vi "Copy of Pulse Train Generation TIO.vi"(8 "error in":errorcluster) -> (0 "error out":errorcluster, 3 "Pulse Generation Task ID's Out":u32[](array[numeric]) format="%.0x")   [LabVIEW 2009]
uses:
  Acquisition Settings.vi
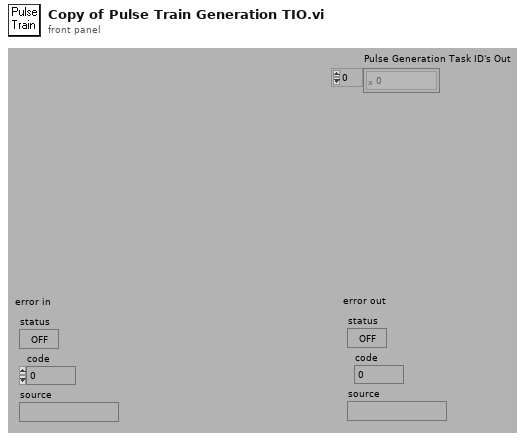
[diagram p1: front panel]
types:
  T1 = cluster{"Name":string, "Device Number":i16, "Counter Number":i16, "Pulse Spec 1 (Clocks)":u32, "Pulse Spec 2 (Clocks)":u32, "Signal Routing Configuration":i16, "Inverted":bool}[]
  T2 = cluster{"Name":string, "Signal Routing":cluster{"signal name":u16, "signal source":u16, "signal source line number":u32, "signal name line number":u32}[]}[]
  T3 = cluster{"Name":string, "Signal Routing":cluster{"signal name":u16, "signal source":u16, "signal source line number":u32, "signal name line number":u32}[]}
  T4 = cluster{"signal name":u16, "signal source":u16, "signal source line number":u32, "signal name line number":u32}[]
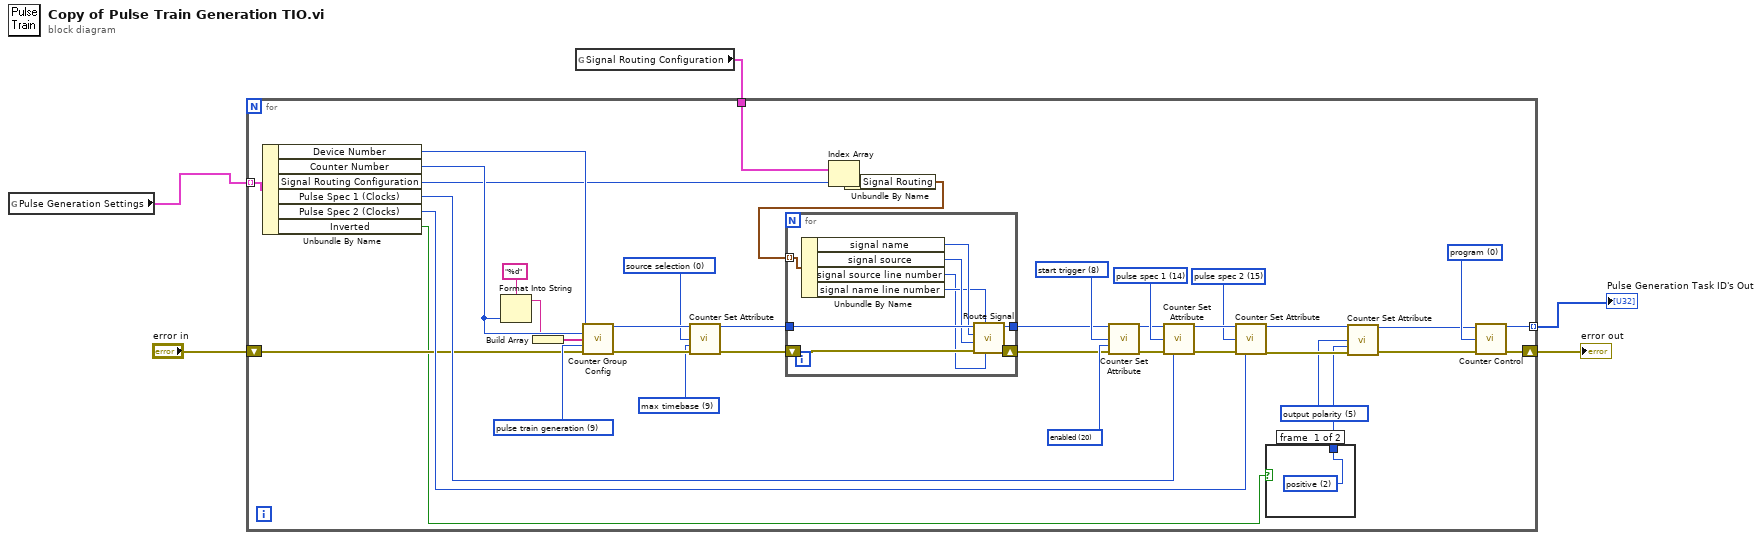
[diagram p0: block diagram]
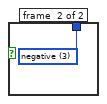
[diagram p2: hidden frame]
diagram:
  n1 = global read "Acquisition Settings.vi" "Pulse Generation Settings"() -> (w2:T1)
  n2 = global read "Acquisition Settings.vi" "Signal Routing Configuration"() -> (w1:T2)
  n3 = for {
    tunnel: w2 -> [w43] mode=indexing
    tunnel: [w42] -> w3 mode=indexing
    shift-right: [w21] -> w4
    shift-left: "error in" -> [w22]
    tunnel: w1 -> [w13]
    w8 = u32 5 items=["source selection", "source polarity", "gate selection", "gate polarity", "output mode", "output polarity", "aux line selection", "aux line polarity", "start trigger", "counting synchronous", "up down", "buffer mode", "encoder type", "initial count", "pulse spec 1", "pulse spec 2", "pulse spec 3", "pulse spec 4", "auto increment", "prescale value", "Z index active", "Z index value", "Z index reload phase", "synchronization line", "synchronization method", "initial seconds", "precision", "transfer method", "start trigger polarity", "timeout", "initial seconds enable"] ("attribute ID")
    w25 = u32 20 items=["yes", "no", "positive", "negative", "high", "low", "low to high", "high to low", "default", "max timebase", "other counter gate", "other counter TC", "other counter output", "other counter source", "source", "gate", "aux line", "in start trigger", "in stop trigger", "automatic", "enabled", "count up", "count down", "hardware", "single", "continuous", "pulse", "toggle", "quadrature encoder X1", "quadrature encoder X2", "quadrature encoder X4", "two pulse counting", "A high B high", "A high B low", "A low B high", "A low B low", "PFI n", "RTSI n", "timebase n", "disabled", "PXI backplane clock", "counter n output", "(Reserved) pulse per second", "(Reserved) IRIG-B", "(Reserved) seconds", "(Reserved) nano seconds", "interrupts", "dma", "RTSI clock"] ("attribute value type")
    w26 = u32 8 items=["source selection", "source polarity", "gate selection", "gate polarity", "output mode", "output polarity", "aux line selection", "aux line polarity", "start trigger", "counting synchronous", "up down", "buffer mode", "encoder type", "initial count", "pulse spec 1", "pulse spec 2", "pulse spec 3", "pulse spec 4", "auto increment", "prescale value", "Z index active", "Z index value", "Z index reload phase", "(Reserved) synchronization line", "(Reserved) synchronization method", "(Reserved) seconds", "(Reserved) precision", "transfer method", "start trigger polarity"] ("attribute ID")
    w29 = u32 9 items=["simple event counting", "single period measurement", "single pulse width measurement", "triggered pulse width measurement", "two signal edge separation measurement", "position measurement", "single pulse generation", "single triggered pulse generation", "retriggerable pulse generation", "pulse train generation", "frequency shift keying", "buffered event counting", "buffered period measurement", "buffered semiperiod measurement", "buffered pulse width measurement", "buffered two signal edge separation measurement", "buffered position measurement"] ("task type")
    w33 = u32 15 items=["source selection", "source polarity", "gate selection", "gate polarity", "output mode", "output polarity", "aux line selection", "aux line polarity", "start trigger", "counting synchronous", "up down", "buffer mode", "encoder type", "initial count", "pulse spec 1", "pulse spec 2", "pulse spec 3", "pulse spec 4", "auto increment", "prescale value", "Z index active", "Z index value"] ("attribute ID")
    w34 = u32 14 items=["source selection", "source polarity", "gate selection", "gate polarity", "output mode", "output polarity", "aux line selection", "aux line polarity", "start trigger", "counting synchronous", "up down", "buffer mode", "encoder type", "initial count", "pulse spec 1", "pulse spec 2", "pulse spec 3", "pulse spec 4", "auto increment", "prescale value", "Z index active", "Z index value"] ("attribute ID")
    w35 = u32 9 items=["yes", "no", "positive", "negative", "high", "low", "low to high", "high to low", "default", "max timebase", "other counter gate", "other counter TC", "other counter output", "other counter source", "source", "gate", "aux line", "in start trigger", "in stop trigger", "automatic", "enabled", "count up", "count down", "hardware", "single", "double", "pulse", "toggle", "quadrature encoder X1", "quadrature encoder X2", "quadrature encoder X4", "two pulse counting", "A high B high", "A high B low", "A low B high", "A low B low", "PFI n", "RTSI n", "timebase n"] ("attribute value type")
    w36 = u32 0 items=["source selection", "source polarity", "gate selection", "gate polarity", "output mode", "output polarity", "aux line selection", "aux line polarity", "start trigger", "counting synchronous", "up down", "buffer mode", "encoder type", "initial count", "pulse spec 1", "pulse spec 2", "pulse spec 3", "pulse spec 4", "auto increment", "prescale value", "Z index active", "Z index value"] ("attribute ID")
    w45 = u32 0 items=["program", "reset", "arm", "prepare", "disarm", "count up", "count down", "switch cycle", "snapshot"] ("control code")
    n4 = Unbundle By Name(w43) -> ("Device Number"=w44:i16, "Counter Number"=w41:i16, "Signal Routing Configuration"=w14:i16, "Pulse Spec 1 (Clocks)"=w24:u32, "Pulse Spec 2 (Clocks)"=w23:u32, "Inverted"=w6:bool)
    n5 = Format Into String(format string="%d" ("Format String"), w41) -> (resulting string=w31:string)  [unwired: 2 in, 1 out]
    n6 = Build Array(w31) -> (w32:string[])
    n7 = call <vilib>:"Counter Group Config.vi"("device"=w44, "group"=w41, "counter list"=w32, "task type"=w29, "error in (no error)"=w22) -> ("task ID"=w40:u32, "error out"=w39:errorcluster)  [unwired: 8 in, 1 out]
    n8 = call <vilib>:"Counter Set Attribute.vi"("task ID in"=w40, "attribute ID"=w36, "attribute value type"=w35, "error in (no error)"=w39) -> ("task ID out"=w18:u32, "error out"=w17:errorcluster)  [unwired: 10 in]
    n9 = Index Array(array=w13, index=w14) -> (element=w19:T3)
    n10 = Unbundle By Name(w19) -> ("Signal Routing"=w20:T4)
    n11 = for {
      tunnel: w18 -> [w56]
      shift-right: [w48] -> w15
      shift-left: w17 -> [w55]
      tunnel: w20 -> [w54] mode=indexing
      tunnel: [w49] -> w16
      n12 = Unbundle By Name(w54) -> ("signal name"=w53:u16, "signal source"=w52:u16, "signal source line number"=w50:u32, "signal name line number"=w51:u32)
      n13 = call <vilib>:"Route Signal.vi"("signal source line number"=w50, "signal name line number"=w51, "error in (no error)"=w55, "signal source"=w52, "signal name"=w53, "task ID"=w56) -> ("error out"=w48:errorcluster, "task ID out"=w49:u32)  [unwired: 4 in]
    }
    n14 = call <vilib>:"Counter Set Attribute.vi"("task ID in"=w16, "attribute ID"=w26, "attribute value type"=w25, "error in (no error)"=w15) -> ("task ID out"=w28:u32, "error out"=w27:errorcluster)  [unwired: 10 in]
    n15 = call <vilib>:"Counter Set Attribute.vi"("task ID in"=w28, "attribute ID"=w34, "error in (no error)"=w27, "attribute value number"=w24) -> ("task ID out"=w38:u32, "error out"=w37:errorcluster)  [unwired: 10 in]
    n16 = call <vilib>:"Counter Set Attribute.vi"("task ID in"=w38, "attribute ID"=w33, "error in (no error)"=w37, "attribute value number"=w23) -> ("task ID out"=w12:u32, "error out"=w11:errorcluster)  [unwired: 10 in]
    n17 = case shown="False" w6 {
      tunnel: [w46 w47] -> w7
      frame #0 {
        w46 = u32 2 items=["yes", "no", "positive", "negative", "high", "low", "low to high", "high to low", "default", "max timebase", "other counter gate", "other counter TC", "other counter output", "other counter source", "source", "gate", "aux line", "in start trigger", "in stop trigger", "automatic", "enabled", "count up", "count down", "hardware", "single", "continuous", "pulse", "toggle", "quadrature encoder X1", "quadrature encoder X2", "quadrature encoder X4", "two pulse counting", "A high B high", "A high B low", "A low B high", "A low B low", "PFI n", "RTSI n", "timebase n", "disabled", "PXI backplane clock", "counter n output", "pulse per second", "IRIG-B", "seconds", "nanoseconds", "interrupts", "dma", "RTSI clock"] ("attribute value type")
      }
      frame #1 {
        w47 = u32 3 items=["yes", "no", "positive", "negative", "high", "low", "low to high", "high to low", "default", "max timebase", "other counter gate", "other counter TC", "other counter output", "other counter source", "source", "gate", "aux line", "in start trigger", "in stop trigger", "automatic", "enabled", "count up", "count down", "hardware", "single", "continuous", "pulse", "toggle", "quadrature encoder X1", "quadrature encoder X2", "quadrature encoder X4", "two pulse counting", "A high B high", "A high B low", "A low B high", "A low B low", "PFI n", "RTSI n", "timebase n", "disabled", "PXI backplane clock", "counter n output", "pulse per second", "IRIG-B", "seconds", "nanoseconds", "interrupts", "dma", "RTSI clock"] ("attribute value type")
      }
    }
    n18 = call <vilib>:"Counter Set Attribute.vi"("task ID in"=w12, "attribute ID"=w8, "attribute value type"=w7, "error in (no error)"=w11) -> ("task ID out"=w10:u32, "error out"=w9:errorcluster)  [unwired: 10 in]
    n19 = call <vilib>:"Counter Control.vi"("task ID"=w10, "control code"=w45, "error in (no error)"=w9) -> ("task ID out"=w42:u32, "error out"=w21:errorcluster)  [unwired: 11 in]
  }
  "error out" <- w4
  "Pulse Generation Task ID's Out" <- w3
